vi "Plot Scales GUI V2.vi"(8 "error in (no error)":errorcluster, 11 "Refs":T6) -> (0 "error out":errorcluster)   [LabVIEW 2021, in "RocketPlot.lvlib"]
uses:
  RocketPlot.lvlib
  TypeDefs/Plot UI references.ctl
  Classes/RocketPlotHandle/RocketPlotHandle.lvclass
  <userlib>/bjustice/TipStripOOPanel/Classes/TipPanelHandle/TipPanelHandle.lvclass
  TypeDefs/Plot top row.ctl
  TypeDefs/Plot axis GUI.ctl
  tick style/plot tick style picture ring.ctl
  lock/plot lock button.ctl
  horiz grid/plot horizontal grid pic ring.ctl
  vert grid/plot vertical grid pic ring.ctl
  <vilib>/Utility/error.llb/Error Cluster From Error Code.vi
  <vilib>/ErrorRing/Error Ring.xnode
  <userlib>/_OpenG.lib/appcontrol/appcontrol.llb/openg_application_control.lvlib
panel:
  in  "X-axis":T1={"Tick Colors:Tick Color"=4294967295, "Tick Colors:Minor Tick Color"=4294967295, "Name Label.Text"="", "Marker Colors:Text Color"=16777225, "Name Label.Font:Size"="", "Marker.Font:Size"="", "Flipped"=FALSE, "Tick Style"=0, "Grid Colors:Major Color"=0, "Grid Colors:Minor Color"=0, "Mapping Mode"=FALSE, "Autoscale?"=FALSE, "Range:Minimum"=0.0, "Range:Maximum"=0.0, "Offset and Multiplier:Multiplier"=0.0, "Offset and Multiplier:Offset"=0.0, "Horiz.Grid Style"=0, "Name Label.Text Colors:Text Color"=0, "Vert.Grid Style"=0, "Name Label.Visible"=FALSE, "Uniform Marker Spacing?"=FALSE, "Format String"=""}
  in  "Title.Visible":bool
  in  "Left axis":T1={"Tick Colors:Tick Color"=4294967295, "Tick Colors:Minor Tick Color"=4294967295, "Name Label.Text"="", "Marker Colors:Text Color"=16777225, "Name Label.Font:Size"="", "Marker.Font:Size"="", "Flipped"=FALSE, "Tick Style"=0, "Grid Colors:Major Color"=0, "Grid Colors:Minor Color"=0, "Mapping Mode"=FALSE, "Autoscale?"=FALSE, "Range:Minimum"=0.0, "Range:Maximum"=0.0, "Offset and Multiplier:Multiplier"=0.0, "Offset and Multiplier:Offset"=0.0, "Horiz.Grid Style"=0, "Name Label.Text Colors:Text Color"=0, "Vert.Grid Style"=0, "Name Label.Visible"=FALSE, "Uniform Marker Spacing?"=FALSE, "Format String"=""}
  in  "Right axis":T1={"Tick Colors:Tick Color"=4294967295, "Tick Colors:Minor Tick Color"=4294967295, "Name Label.Text"="", "Marker Colors:Text Color"=16777225, "Name Label.Font:Size"="", "Marker.Font:Size"="", "Flipped"=FALSE, "Tick Style"=0, "Grid Colors:Major Color"=0, "Grid Colors:Minor Color"=0, "Mapping Mode"=FALSE, "Autoscale?"=FALSE, "Range:Minimum"=0.0, "Range:Maximum"=0.0, "Offset and Multiplier:Multiplier"=0.0, "Offset and Multiplier:Offset"=0.0, "Horiz.Grid Style"=0, "Name Label.Text Colors:Text Color"=0, "Vert.Grid Style"=0, "Name Label.Visible"=FALSE, "Uniform Marker Spacing?"=FALSE, "Format String"=""}
  in  "Title":string
  in  "Plot Area:Colors:BG Color":u32(colorbox) caption="Plot area color"
  in  "Cancel":bool
  in  "Apply":bool
  # "General"
  # "X-axis"
  # "Left\nY-axis"
  # "Right\nY-axis"
  # "Scaling Factors"
  # "Font Sizes"
  # "Scaling Factors"
  # "Font Sizes"
  # "Scaling Factors"
  # "Font Sizes"
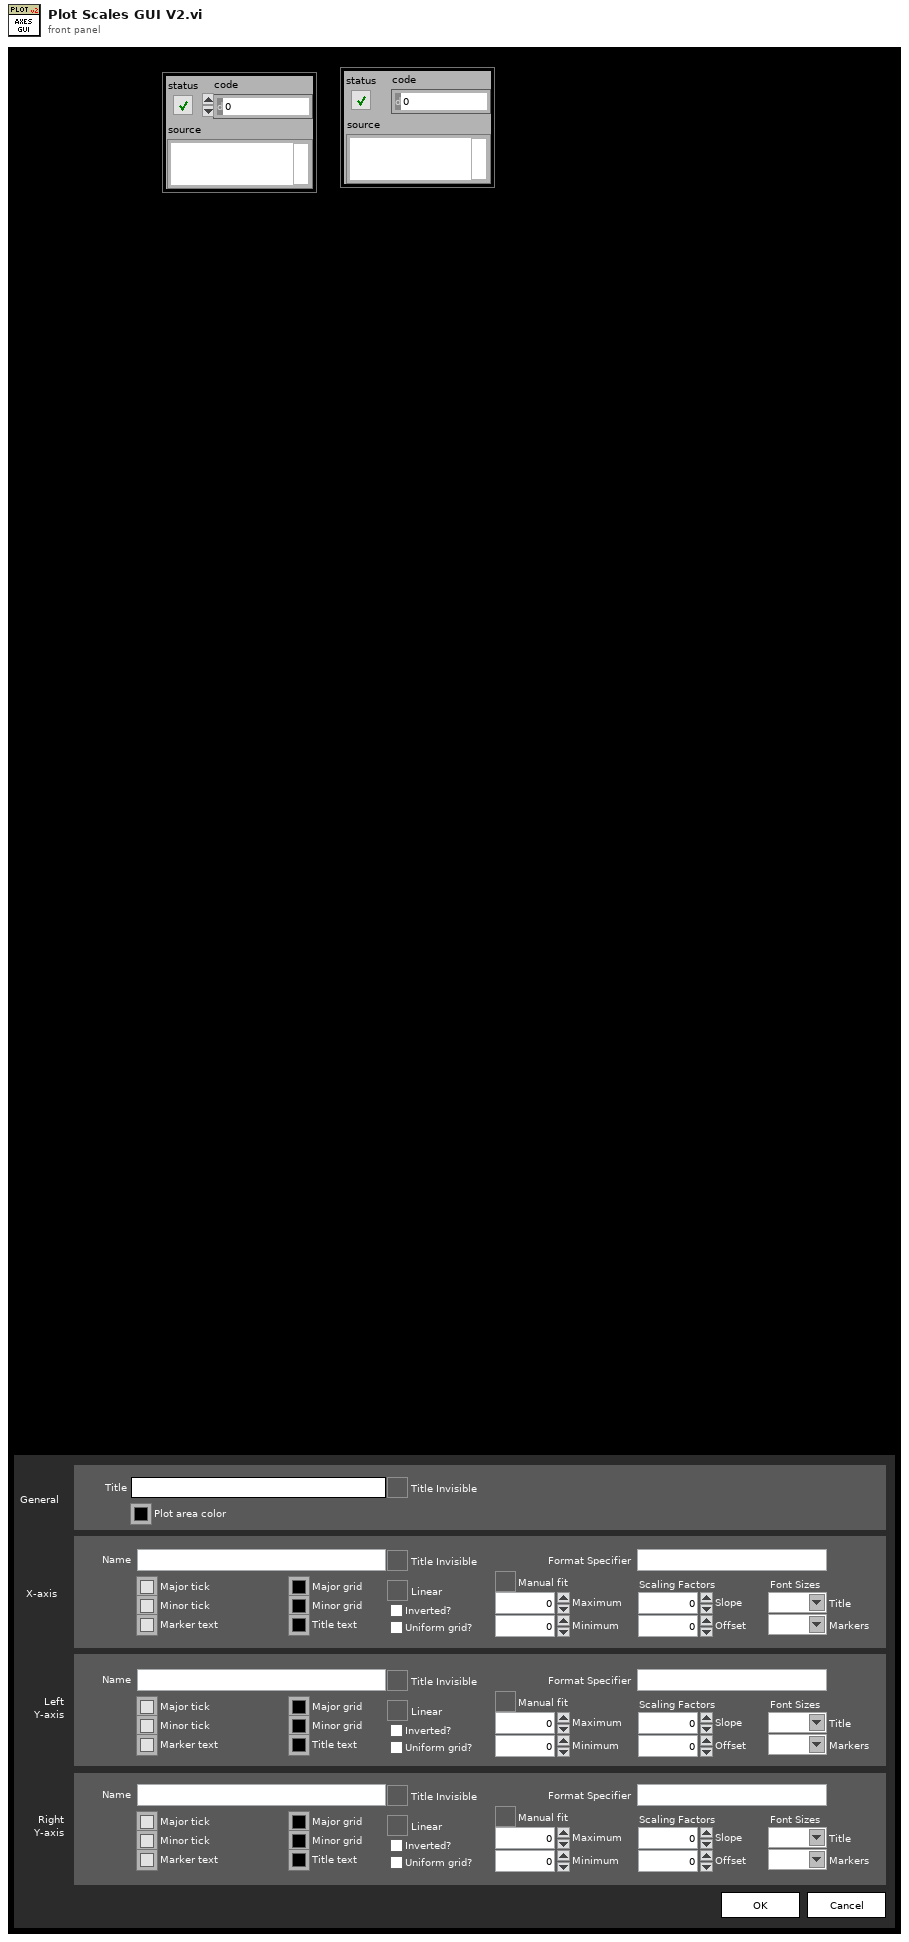
[diagram p1: front panel]
types:
  T1 = typedef "RocketPlot.lvlib/Plot axis GUI.ctl" = cluster{"Tick Colors:Tick Color":u32, "Tick Colors:Minor Tick Color":u32, "Name Label.Text":string, "Marker Colors:Text Color":u32, "Name Label.Font:Size":string, "Marker.Font:Size":string, "Flipped":bool, "Tick Style":T2, "Grid Colors:Major Color":u32, "Grid Colors:Minor Color":u32, "Mapping Mode":bool, "Autoscale?":T3, "Range:Minimum":dbl, "Range:Maximum":dbl, "Offset and Multiplier:Multiplier":dbl, "Offset and Multiplier:Offset":dbl, "Horiz.Grid Style":T4, "Name Label.Text Colors:Text Color":u32, "Vert.Grid Style":T5, "Name Label.Visible":bool, "Uniform Marker Spacing?":bool, "Format String":string}
  T2 = typedef "RocketPlot.lvlib/plot tick style picture ring.ctl" = u16
  T3 = typedef "RocketPlot.lvlib/plot lock button.ctl" = bool
  T4 = typedef "RocketPlot.lvlib/plot horizontal grid pic ring.ctl" = u16
  T5 = typedef "RocketPlot.lvlib/plot vertical grid pic ring.ctl" = u16
  T6 = typedef "RocketPlot.lvlib/Plot UI references.ctl" = cluster{"Title":refnum<vi>, "Title?":refnum<vi>, "Visible sidebar?":refnum<vi>, "Time to Plot":refnum<vi>, "top array":refnum<vi>, "Scrollbar":refnum<vi>, "tab ref":refnum<vi>, "Add row":refnum<vi>, "TopArray":cluster{"PID":refnum<vi>, "Numeric color":refnum<vi>, "Flat":refnum<vi>, "PID color":refnum<vi>, "Data":refnum<vi>}, "Splitter":refnum<vi>, "Front Panel":refnum<vi>, "VI":refnum<vi>, "Meta LUT":refnum<data-value>, "spoof":refnum<vi>, "BluePlotHandle":refnum<class "RocketPlotHandle.lvclass">, "PlotPane":refnum<vi>, "X Scale":refnum<vi>, "Left Scale":refnum<vi>, "Right Scale":refnum<vi>, "TimeZone":refnum<vi>, "ShowPlotToolBar":refnum<vi>, "DeferResize?":refnum<vi>, "LegendPane":refnum<vi>, "Plot":refnum<vi>, "PlotToolBar":refnum<vi>, "TB.Info":refnum<vi>, "TB.max":refnum<vi>, "X Scale.Plot Name":refnum<vi>, "X Scale.Use Plot Name?":refnum<vi>, "TipPanel":refnum<class "TipPanelHandle.lvclass">}
  T7 = enum32{"Invalid", "Standard", "Closed", "Hidden", "Minimized", "Maximized"}
  T8 = typedef "RocketPlot.lvlib/plot load data V2.ctl" = cluster{"plots":T9[], "X-axis":T11, "Y-axes":T11[], "General":T12}
  T9 = typedef "RocketPlot.lvlib/plot properties V2.ctl" = cluster{"attributes":T10, "Numeric":dbl, "Flatline?":bool}
  T10 = typedef "RocketPlot.lvlib/plot attributes V2.ctl" = cluster{"Plot Color":u32, "Point Style":u8, "Line Style":u8, "Plot Interpolation":u8, "Line Width":u8, "Bar Plot Style":u8, "Fill To":i16, "X Scale Index":u32, "Y Scale Index":u32, "Anti-aliased":bool, "Label Format":u8, "Digital Transition Type":u8, "Digital Transition Location":u8, "Digital Line Style":u8, "Fill/Point Color":u32, "Plot Name":string, "Visible":bool}
  T11 = typedef "RocketPlot.lvlib/Plot scale axis properties.ctl" = cluster{"Name Label.Text":string, "Style":u8, "Tick Colors:Minor Tick Color":u32, "Tick Colors:Tick Color":u32, "Marker Colors:Text Color":u32, "Grid Colors:Major Color":u32, "Grid Colors:Minor Color":u32, "Mapping Mode":u8, "Flipped":bool, "Name Label.Visible":bool, "Name Label.Text Colors:Text Color":u32, "Scale Fit":u8, "Range:Maximum":dbl, "Range:Minimum":dbl, "Offset and Multiplier:Multiplier":dbl, "Offset and Multiplier:Offset":dbl, "Name Label.Font:Size":u32, "Marker.Font:Size":u32, "Uniform Marker Spacing?":bool, "Format String":string}
  T12 = typedef "RocketPlot.lvlib/Plot general properties.ctl" = cluster{"Title":string, "Time to Plot":dbl, "Title.Visible":bool, "Sidebar.Visible":bool, "Plot Area:Colors:BG Color":u32, "X Scale.Plot Name":string, "X Scale.Use Plot Name":bool}
  T13 = typedef "RocketPlot.lvlib/Plot axis gui refs.ctl" = cluster{"Range:Maximum":refnum<vi>, "Range:Minimum":refnum<vi>}
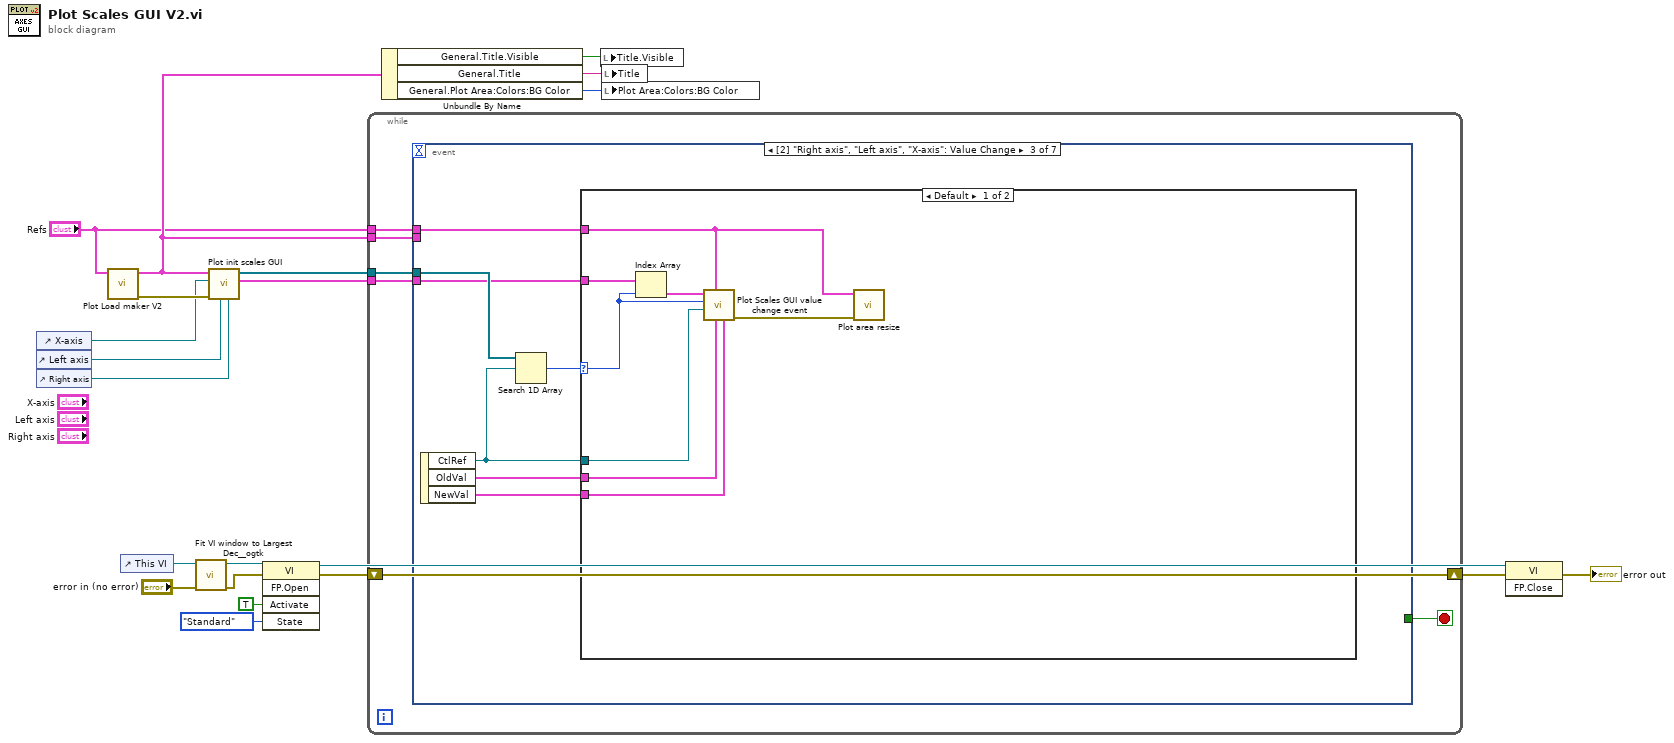
[diagram p0: block diagram]
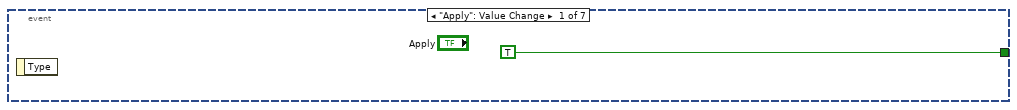
[diagram p2: hidden frame]
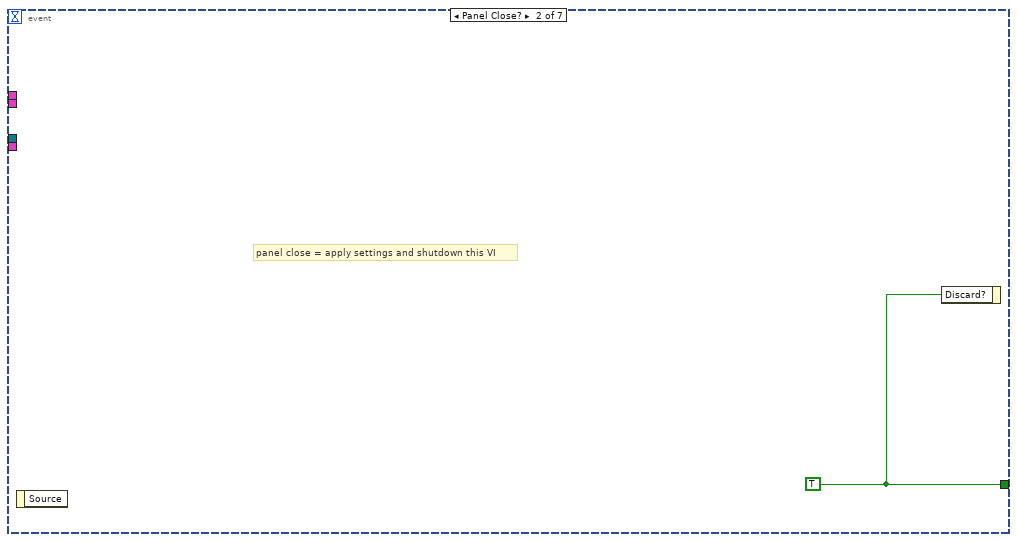
[diagram p3: hidden frame]
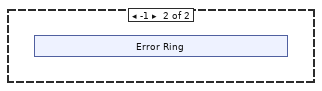
[diagram p4: hidden frame]
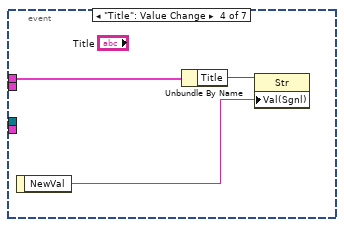
[diagram p5: hidden frame]
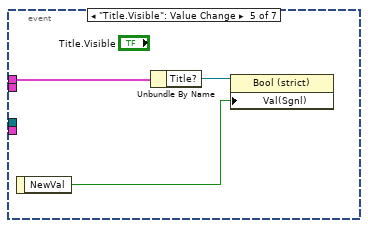
[diagram p6: hidden frame]
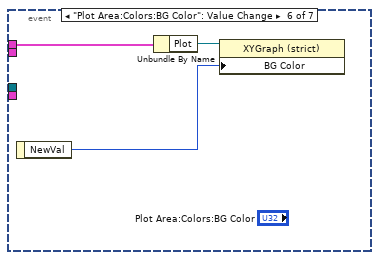
[diagram p7: hidden frame]
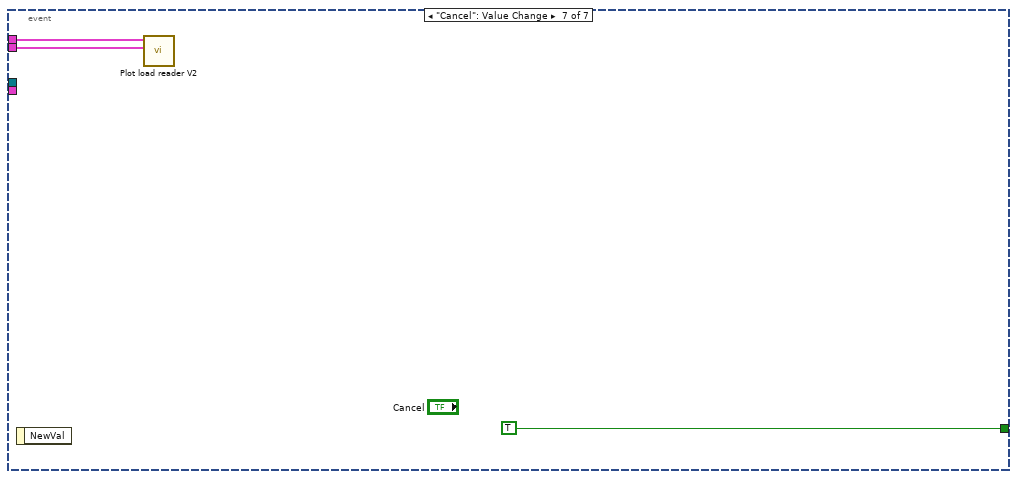
[diagram p8: hidden frame]
diagram:
  n1 = control-ref of="X-axis"() -> (w9:refnum<vi>)
  n2 = control-ref of="Left axis"() -> (w8:refnum<vi>)
  n3 = control-ref of="Right axis"() -> (w7:refnum<vi>)
  n4 = call "Plot Load maker V2.vi"("Refs"="Refs") -> ("error out"=w10:errorcluster, "Plot config"=w4:T8)  [unwired: 9 in]
  n5 = control-ref of="This VI"() -> (w21:refnum<vi>)
  n6 = call <userlib>:"Fit VI window to Largest Dec__ogtk.vi"("error in (no error)"="error in (no error)", "VI Ref (calling VI)"=w21) -> ("error out"=w15:errorcluster, "dup VI Ref"=w17:refnum<vi>)  [unwired: 4 in]
  n7 = call "Plot init scales GUI.vi"("Right axis"=w7, "Left axis"=w8, "error in (no error)"=w10, "X-axis"=w9, "Plot config"=w4) -> ("axis SubRefs"=w5:T13[], "Axis references"=w6:refnum<vi>[])  [unwired: 4 in, 1 out]
  n8 = invoke class="VI" method="FP.Open"(reference=w17, error in=w15, "Activate"=TRUE ("Activate?"), "State"=T7."Standard") -> (reference out=w3:refnum<vi>, error out=w2:errorcluster)  [unwired: 1 in, 3 out]
  n9 = while {
    shift-right: [w26] -> w14
    shift-left: w2 -> [w26]
    tunnel: w6 -> [w25]
    tunnel: w5 -> [w24]
    tunnel: "Refs" -> [w23]
    tunnel: w4 -> [w22]
    stop <- w27 stop-if-true
    n10 = event shown="[2] \"Right axis\", \"Left axis\", \"X-axis\": Value Change" {
      selector: _ -> [_ _ _ _ _ _ _]
      dyn-events: _ -> [_ _ _ _ _ _ _]
      timeout: _ -> [_ _ _ _ _ _ _]
      tunnel: [TRUE w29 _ _ _ _ TRUE] -> w27
      tunnel: w25 -> [_ _ w36 _ _ _ _]
      tunnel: w24 -> [_ _ w34 _ _ _ _]
      tunnel: w23 -> [_ _ w32 w52 w55 w58 w60]
      tunnel: w22 -> [_ _ _ _ _ _ w59]
      event "Apply": Value Change {
        n11 = event-data() -> ()  [unwired: 1 in, 1 out]
      }
      event Panel Close? {
        w29 = TRUE
        # "panel close = apply settings and shutdown this VI"
        n12 = event-data() -> ()  [unwired: 1 in, 1 out]
        n13 = event-data("Discard?"=w29) -> ()  [unwired: 1 in, 1 out]
      }
      event Value Change {
        n14 = event-data() -> ("CtlRef"=w33:refnum<vi>, "OldVal"=w31:T1, "NewVal"=w30:T1)  [unwired: 1 in]
        n15 = Search 1D Array(1D array=w36, element=w33) -> (index of element=w35:i32)  [unwired: 1 in]
        n16 = case shown="Default" w35 {
          selector: w35 -> [w40 _]
          tunnel: w34 -> [w44 _]
          tunnel: w33 -> [w39 _]
          tunnel: w32 -> [w38 _]
          tunnel: w31 -> [w42 _]
          tunnel: w30 -> [w41 _]
          frame Default {
            n17 = Index Array(array=w44, index=w40) -> (element=w43:T13)
            n18 = call "Plot Scales GUI value change event.vi"("NewVal"=w41, "OldVal"=w42, "Refs"=w38, "Axis reference"=w39, "Index"=w40, "axis SubRefs"=w43) -> ("error out"=w37:errorcluster)  [unwired: 5 in]
            n19 = call "Plot area resize.vi"("error in (no error)"=w37, "Refs"=w38) -> ()  [unwired: 9 in, 1 out]
          }
          frame -1 {
            n20 = xnode "Error Ring"() -> ()  [unwired: 1 out]
          }
        }
      }
      event "Title": Value Change {
        n21 = event-data() -> ("NewVal"=w50:string)  [unwired: 1 in]
        n22 = Unbundle By Name(w52) -> ("Title"=w51:refnum<vi>)
        n23 = property class="Str"(reference=w51, "Val(Sgnl)"=w50) -> ()  [unwired: 1 in, 2 out]
      }
      event "Title.Visible": Value Change {
        n24 = event-data() -> ("NewVal"=w53:bool)  [unwired: 1 in]
        n25 = Unbundle By Name(w55) -> ("Title?"=w54:refnum<vi>)
        n26 = property class="Bool (strict)"(reference=w54, "Val(Sgnl)"=w53) -> ()  [unwired: 1 in, 2 out]
      }
      event "Plot Area:Colors:BG Color": Value Change {
        n27 = event-data() -> ("NewVal"=w56:u32)  [unwired: 1 in]
        n28 = Unbundle By Name(w58) -> ("Plot"=w57:refnum<vi>)
        n29 = property class="XYGraph (strict)"(reference=w57, "BG Color"=w56) -> ()  [unwired: 1 in, 2 out]
      }
      event "Cancel": Value Change {
        n30 = event-data() -> ()  [unwired: 1 in, 1 out]
        n31 = call "Plot load reader V2.vi"("Plot config"=w59, "Refs"=w60) -> ()  [unwired: 9 in, 1 out]
      }
    }
  }
  n32 = Unbundle By Name(w4) -> ("General.Title.Visible"=w11:bool, "General.Title"=w12:string, "General.Plot Area:Colors:BG Color"=w13:u32)
  n33 = local write "Title.Visible"(w11) -> ()
  n34 = local write "Title"(w12) -> ()
  n35 = local write "Plot Area:Colors:BG Color"(w13) -> ()
  n36 = invoke class="VI" method="FP.Close"(reference=w3, error in=w14) -> (error out=→"error out":errorcluster)  [unwired: 1 in, 2 out]
